vi "Write.vi"(8 "error in (no error)":errorcluster, 9 "timeout ms (5000)":i32=5000, 10 "Bytes to write":u8[](array[numeric]), 11 "OpenSSL Socket in":refnum<class "SSL Socket.lvclass">) -> (0 "error out":errorcluster, 2 "bytes written":i32, 3 "OpenSSL Socket out":refnum<class "SSL Socket.lvclass">)   [LabVIEW 2013, in "OpenSSL Socket.lvlib" / "SSL Socket.lvclass"]
doc: "Writes data to the socket."
uses:
  SSL Socket.lvclass
  SSL Socket.lvclass/SSL Socket.ctl
  SSL_Lib/BIO/BIO.lvclass
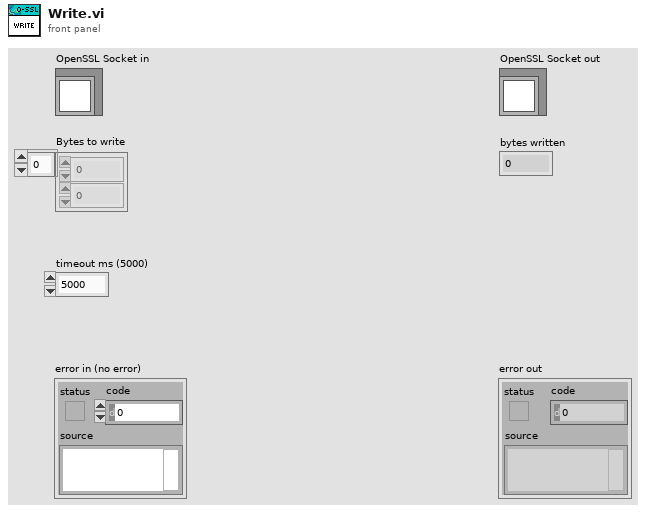
[diagram p1: front panel]
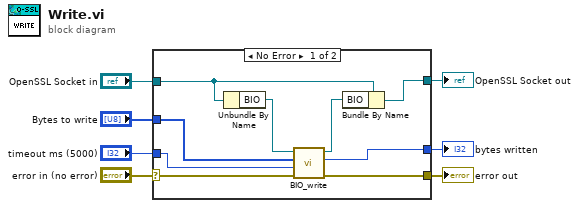
[diagram p0: block diagram]
diagram:
  n1 = case shown="No Error" "error in (no error)" {
    selector: "error in (no error)" -> [w9 w17]
    tunnel: [w16 w17] -> w7
    tunnel: "Bytes to write" -> [w15 _]
    tunnel: "timeout ms (5000)" -> [w8 _]
    tunnel: "OpenSSL Socket in" -> [w13 w18]
    tunnel: [w11 w18] -> w3
    tunnel: [w10 _] -> w2
    frame No Error {
      n2 = Unbundle By Name(w13) -> ("BIO"=w14:refnum<class "BIO.lvclass">)
      n3 = call "BIO_write.vi"("error in (no error)"=w9, "Timeout (10000ms)"=w8, "Bytes to write"=w15, "BIO in"=w14) -> ("error out"=w16:errorcluster, "Bytes written"=w10:i32, "BIO out"=w12:refnum<class "BIO.lvclass">)  [unwired: 5 in]
      n4 = Bundle By Name(cluster=w13, "BIO"=w12) -> (w11:refnum<class "SSL Socket.lvclass">)
    }
    frame Error {
    }
  }
  "error out" <- w7
  "OpenSSL Socket out" <- w3
  "bytes written" <- w2
